vi "UDS_Create.vi"(0 "reference in":refnum<class "UDS.lvclass">, 5 "error in (no error)":errorcluster) -> (14 "reference out":refnum<class "UDS.lvclass">, 19 "error out":errorcluster)   [LabVIEW 2020, in "ECU_Diagnose.lvlib" / "UDS.lvclass"]
doc: "Constructor."
uses:
  UDS.lvclass
  C:/Program Files (x86)/National Instruments/LabVIEW 2020/vi.lib/addons/_AddQ/G#Object/G#Object.lvclass
  <vilib>/addons/_AddQ/G#Object/G#Object.lvclass
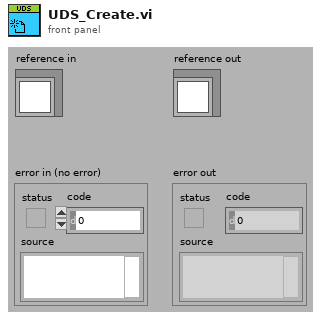
[diagram p1: front panel]
types:
  T1 = typedef "ECU_Diagnose.lvlib/UDS.lvclass/ObjectAttributesRef.ctl" = refnum<data-value>
  T2 = typedef "ECU_Diagnose.lvlib/UDS.lvclass/ObjectAttributes.ctl" = cluster{"MyAttribute":dbl, "UDSSetting":cluster{"InterfacName":string, "Baud Rate":u64, "FD Baud Rate":u64, "Transport Protocol":T3, "IO Mode":u32, "Max DLC":u16, "Transmit ID":u32, "Receive ID":u32, "Wait Time CF (STmin)":u32, "Fill Byte":u32}, "diag ref":T4}
  T3 = typedef "NI_Automotive Diagnostic Command Set.lvlib/Transport Protocol Selector.ctl" = enum16{"ISO TP - Normal Mode", "ISO TP - Mixed Mode", "VW TP 2.0", "Diagnostics on IP", "ISO TP LIN"}
  T4 = typedef "NI_Automotive Diagnostic Command Set.lvlib/Diag Reference.ctl" = cluster{"Diag CAN Handle":u32, "Transport Protocol":T3, "Receive Address Extension":u8, "Transmit Address Extension":u8, "Receive CAN Id":u32, "Transmit CAN Id":u32, "Log Frames ?":bool, "My TP Address":u8, "Other TP Address":u8, "T1":u16, "T2":u16, "T3":u16, "T4":u16, "Tx SN":u8, "Block Size":u8, "Rx SN":u8, "VW TP Initialized?":bool, "Tx block no":u8, "baud rate":u64, "Interface":string, "Channel Diag CAN Handle":u32, "UDP Connection ID":refnum<k16>, "TCP Connection ID":refnum<k5>, "Target IP Addr":u32, "Source Address":u16, "Target Address":u16, "Send Header NACK?":bool, "DLL Handle":u32, "NAD":u8, "Time Stamp read first":dbl, "Time Stamp read last":dbl, "Time Stamp write first":dbl, "Time Stamp write last":dbl, "Time Stamp write":dbl, "Time Stamp read":dbl, " I/O Mode":u32, "FD Baudrate":u64, "TX_DL":u16, "RX_DL":u16, "DoIP Protocol Version":T5, " Selected I/O Mode":u32, "TesterPresent Counter":u32, "TesterPresent Limit":u32, "TesterPresent Tick[ms]":i32, "TesterPresent RequireResponse?":bool, "TesterPresent Stored Ref?":bool, "TesterPresent Message":u8[], "TesterPresent Task Handle":i32, "TesterPresent Semaphore":T6, "Response Plausibility Check":u32, "Default Version?":bool, "Diagostic Globals":T7, "Session-based Properties?":bool}
  T5 = typedef "NI_Automotive Diagnostic Command Set.lvlib/DoIP Protocol Version.ctl" = u8
  T6 = typedef "Semaphore RefNum" = refnum<k1>
  T7 = typedef "NI_Automotive Diagnostic Command Set.lvlib/Diag Globals.ctl" = cluster{"Timeout FC (Bs)":u32, "Timeout CF (Cr)":u32, "Timeout Diag Command":u32, "Receive Block Size (BS)":u8, "Wait Time CF (STmin)":u8, "Max Waits (N_WFTmax)":u8, "Waits to Send (N_WAIT)":i32, "Time between Waits (TW)":u32, "Fill CAN Frames?":bool, "Fill Byte":u32, "Invalid Response as Error?":bool, "Max RspPending Count":u32, "VWTP Command Timeout":u32, "Transport Protocol":T3, "Diag CAN Handle":u32, "DLL Handle":u32, "Timeout RspPending":u32}
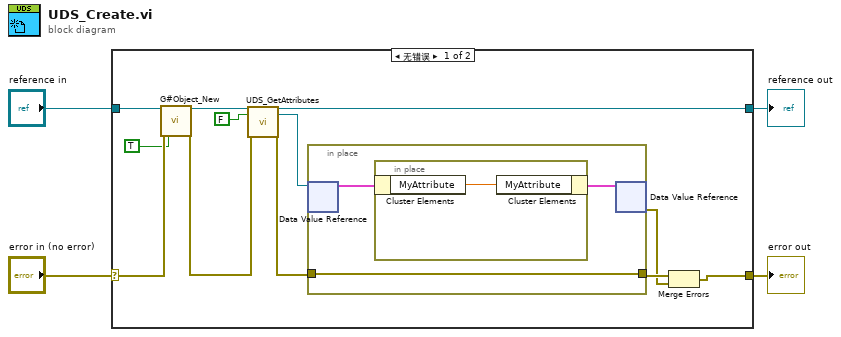
[diagram p0: block diagram]
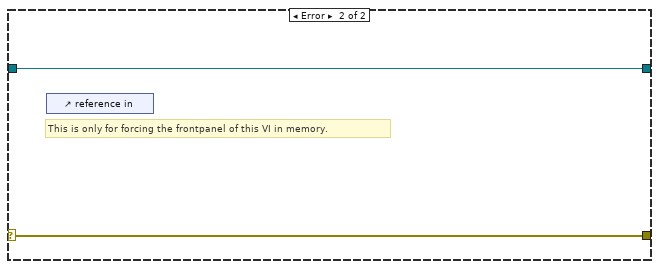
[diagram p2: hidden frame]
diagram:
  n1 = case shown="无错误" "error in (no error)" {
    selector: "error in (no error)" -> [w15 w22]
    tunnel: [w14 w22] -> w3
    tunnel: [w9 w21] -> w1
    tunnel: "reference in" -> [w16 w21]
    frame No Error {
      n2 = call <vilib>:"G#Object_New.vi"("reference in"=w16, "error in (no error)"=w15, "user counter (T)?"=TRUE ("User Counter")) -> ("reference out"=w10:refnum<class "UDS.lvclass">, "error out"=w8:errorcluster)  [unwired: 14 in, 1 out]
      n3 = call "UDS_GetAttributes.vi"("reference in"=w10, "return data? (T)"=FALSE ("return data"), "error in (no error)"=w8) -> ("reference out"=w9:refnum<class "UDS.lvclass">, "attributes ref"=w6:T1, "error out"=w7:errorcluster)  [unwired: 13 in, 1 out]
      n4 = in-place {
        in-place-border: w7 -> [w17]
        in-place-border: [w17] -> w12
        n5 = in-place-dvr #1(w6) -> (w18:T2)  [unwired: 1 out]
        n6 = in-place {
          n7 = in-place-cluster #2(w18) -> ("MyAttribute"=w20:dbl)
          n8 = in-place-cluster #2("MyAttribute"=w20) -> (w19:T2)
        }
        n9 = in-place-dvr #1(w19) -> (w11:errorcluster)  [unwired: 1 out]
      }
      n10 = Merge Errors(w12, w11) -> (w14:errorcluster)
    }
    frame Error {
      # "This is only for forcing the frontpanel of this VI in memory."
      n11 = control-ref of="reference in"() -> ()  [unwired: 1 out]
    }
  }
  "error out" <- w3
  "reference out" <- w1
